vi "DTC_PERSISTANT.vi"(8 "errin":errorcluster, 11 "UNINIT?":bool) -> (0 "error out":errorcluster, 3 "Erased?":bool)   [LabVIEW 2020]
uses:
  <userlib>/PCAN Basic/Controls/BaudrateEenum.ctl
  <userlib>/PCAN Basic/Controls/Channel.ctl
  41182dc3-e488-4534-8057-e389c647f1e6.vi
  OP500/VG/VG_branche.vi
  <userlib>/Alex_Peak_lib/PEAK_lib_ALEX.lvlib
  <userlib>/PCAN Basic/PCANBasic.lvlib
panel:
  out "dataout":T1 {"ID" format="%.0x"}
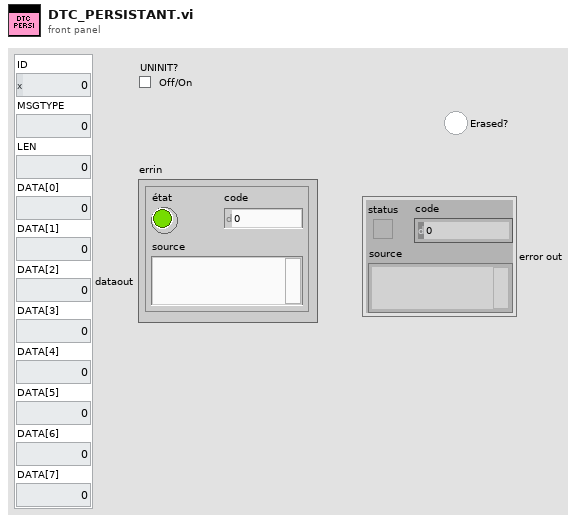
[diagram p1: front panel]
types:
  T1 = cluster{"ID":u32, "MSGTYPE":u8, "LEN":u8, "DATA[0]":u8, "DATA[1]":u8, "DATA[2]":u8, "DATA[3]":u8, "DATA[4]":u8, "DATA[5]":u8, "DATA[6]":u8, "DATA[7]":u8}
  T2 = typedef "PCANBasic.lvlib/Channel.ctl" = enum16{"PCAN_NONEBUS", "not used1", "not used2", "not used3", "not used4", "not used5", "not used6", "not used7", "not used8", "not used9", "not used10", "not used11", "not used12", "not used13", "not used14", "not used15", "not used16", "not used17", "not used18", "not used19", "not used20", "not used21", "not used22", "not used23", "not used24", "not used25", "not used26", "not used27", "not used28", "not used29", "not used30", "not used31", "not used32", "PCAN_ISABUS1", "PCAN_ISABUS2", "PCAN_ISABUS3", "PCAN_ISABUS4", "PCAN_ISABUS5", "PCAN_ISABUS6", "PCAN_ISABUS7", "PCAN_ISABUS8", "not used41", "not used42", "not used43", "not used44", "not used45", "not used46", "not used47", "not used48", "PCAN_DNGBUS1", "not used50", "not used51", "not used52", "not used53", "not used54", "not used55", "not used56", "not used57", "not used58", "not used59", "not used60", "not used61", "not used62", "not used63", "not used64", "PCAN_PCIBUS1", "PCAN_PCIBUS2", "PCAN_PCIBUS3", "PCAN_PCIBUS4", "PCAN_PCIBUS5", "PCAN_PCIBUS6", "PCAN_PCIBUS7", "PCAN_PCIBUS8", "not used73", "not used74", "not used75", "not used76", "not used77", "not used78", "not used79", "not used80", "PCAN_USBBUS1", "PCAN_USBBUS2", "PCAN_USBBUS3", "PCAN_USBBUS4", "PCAN_USBBUS5", "PCAN_USBBUS6", "PCAN_USBBUS7", "PCAN_USBBUS8", "Not used89", "Not used90", "Not used91", "Not used92", "Not used93", "Not used94", "Not used95", "Not used96", "PCAN_PCCBUS1", "PCAN_PCCBUS2"}
  T3 = typedef "PCANBasic.lvlib/BaudrateEenum.ctl" = enum16{"CAN_Baud_1M", "CAN_Baud_800K", "CAN_BAUD_500K", "CAN_BAUD_250K", "CAN_BAUD_125K", "CAN_BAUD_100K", "CAN_BAUD_95K", "CAN_BAUD_83K", "CAN_BAUD_50K", "CAN_BAUD_47K", "CAN_BAUD_33K", "CAN_BAUD_20K", "CAN_BAUD_10K", "CAN_BAUD_5K", "User Baudrate"}
  T4 = cluster{"ID":u32, "MSGTYPE":u8, "LEN":u8, "DATA[0]":ext, "DATA[1]":ext, "DATA[2]":ext, "DATA[3]":ext, "DATA[4]":ext, "DATA[5]":ext, "DATA[6]":ext, "DATA[7]":ext}
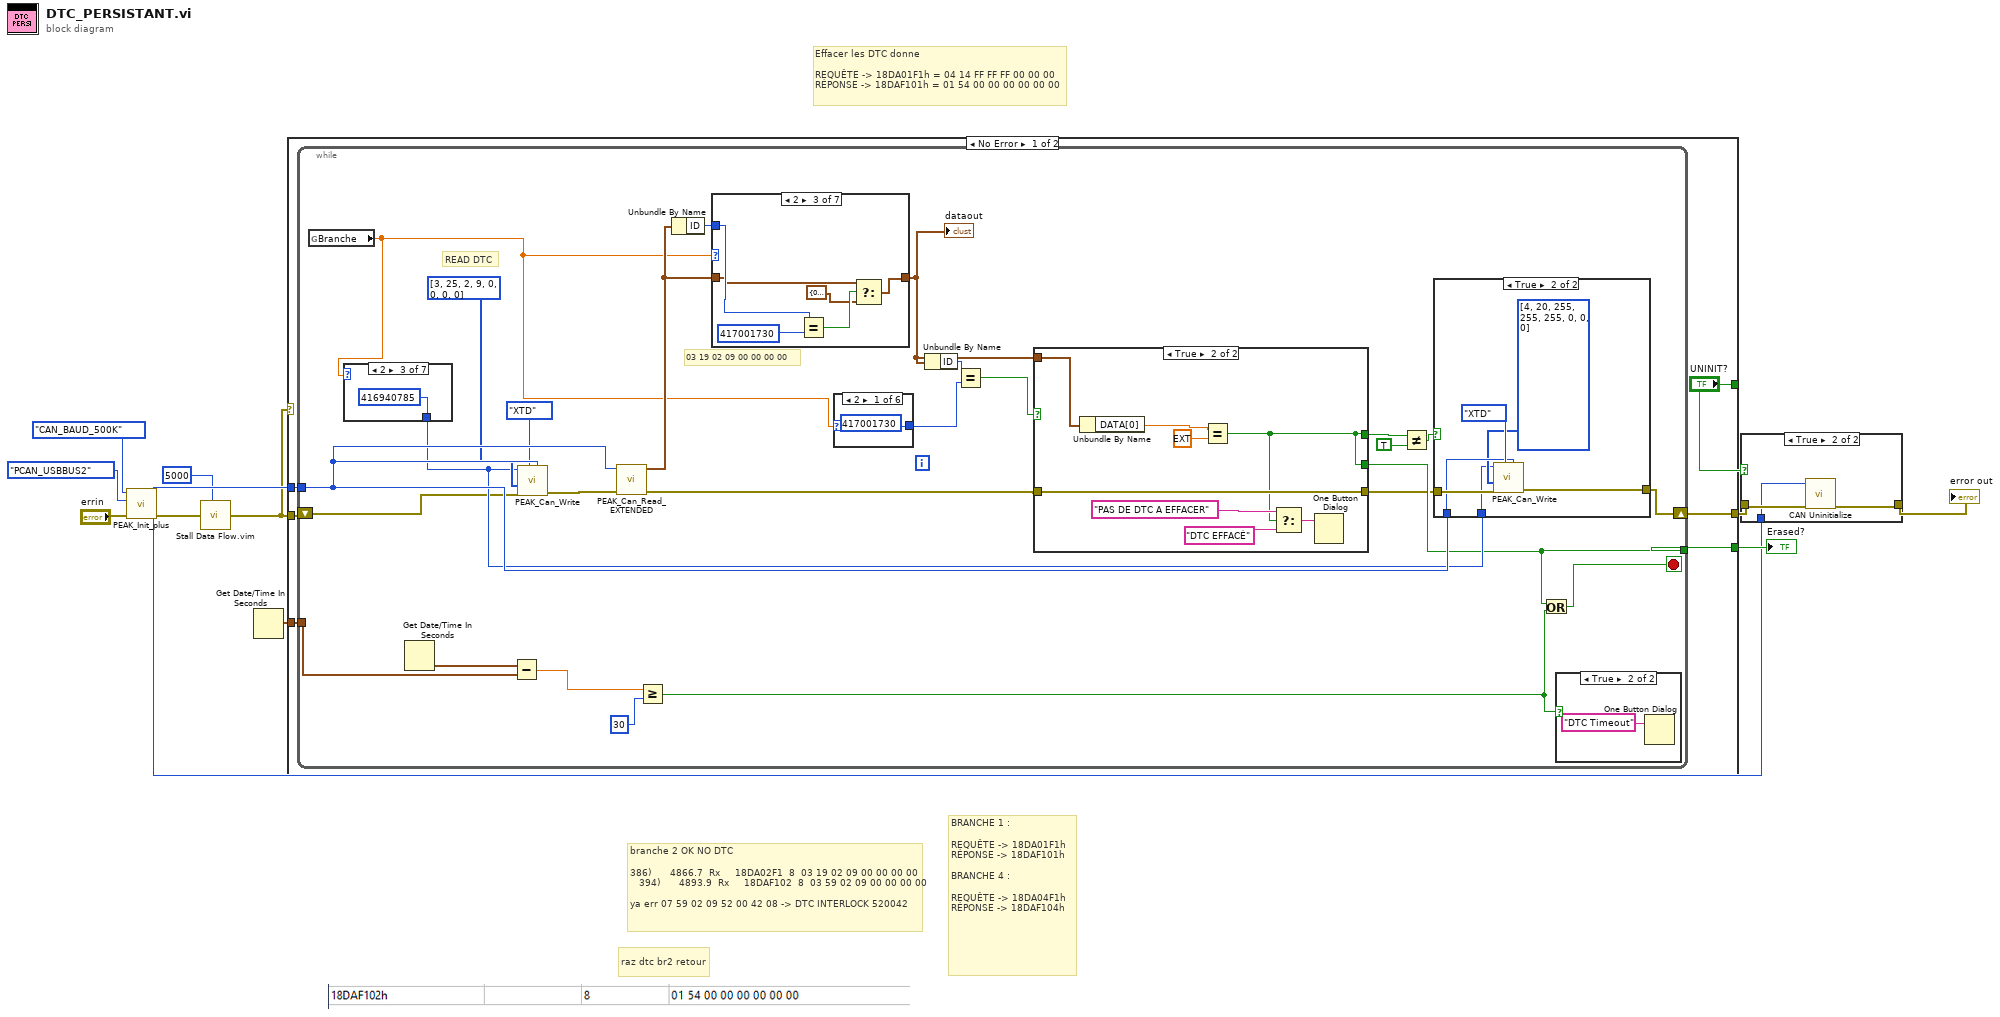
[diagram p0: block diagram]
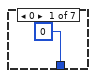
[diagram p2: hidden frame]
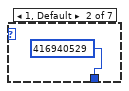
[diagram p3: hidden frame]
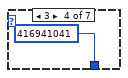
[diagram p4: hidden frame]
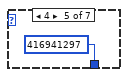
[diagram p5: hidden frame]
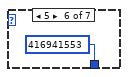
[diagram p6: hidden frame]
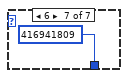
[diagram p7: hidden frame]
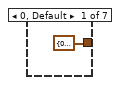
[diagram p8: hidden frame]
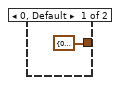
[diagram p10: hidden frame]
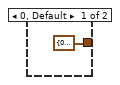
[diagram p12: hidden frame]
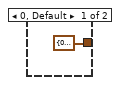
[diagram p14: hidden frame]
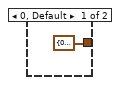
[diagram p16: hidden frame]
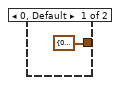
[diagram p18: hidden frame]
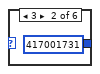
[diagram p19: hidden frame]
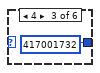
[diagram p20: hidden frame]
diagram:
  # "raz dtc br2 retour"
  # "branche 2 OK NO DTC\n\n386)      4866.7  Rx     18DA02F1  8  03 19 02 09 00 00 00 00 \n   394)      4893.9  Rx     18DAF102  8  03 59 02 09 00 00 00 00\n\nya err 07 59 02 09 52 00 42 08 -> DTC INTERLOCK 520042"
  # "BRANCHE 1 :\n\nREQUÊTE -> 18DA01F1h\nRÉPONSE -> 18DAF101h\n\nBRANCHE 4 :\n\nREQUÊTE -> 18DA04F1h\nRÉPONSE -> 18DAF104h"
  # "Effacer les DTC donne \n\nREQUÊTE -> 18DA01F1h = 04 14 FF FF FF 00 00 00\nRÉPONSE -> 18DAF101h = 01 54 00 00 00 00 00 00"
  n1 = call <userlib>:"PEAK_Init_plus.vi"("errin"="errin", "Channel"=Channel."PCAN_USBBUS2", "BTR0BTR1"=BaudrateEenum."CAN_BAUD_500K") -> ("errout"=w3:errorcluster, "Channel out"=w4:T2)  [unwired: 7 in]
  n2 = call "Stall Data Flow.vim"("value in"=w3, "milliseconds to wait"=u32 5000) -> ("value out"=w2:errorcluster)  [unwired: 1 out]
  n3 = Get Date/Time In Seconds() -> (seconds since 1Jan1904=w10:timestamp)
  n4 = case shown="No Error" w2 {
    tunnel: w2 -> [w18 w109]
    tunnel: [w17 _] -> w11
    tunnel: w10 -> [w16 _]
    tunnel: [w15 w109] -> w9
    tunnel: ["UNINIT?" FALSE ("UNINIT?")] -> w7
    tunnel: w4 -> [w13 _]
    frame No Error {
      n5 = while {
        tunnel: w13 -> [w41]
        shift-right: [w33] -> w15
        shift-left: w18 -> [w30]
        tunnel: [w28] -> w17
        tunnel: w16 -> [w27]
        stop <- w29 stop-if-true
        # "READ DTC"
        # "03 19 02 09 00 00 00 00"
        n6 = global read "VG_branche.vi" "Branche"() -> (w31:dbl)
        n7 = case shown="2" w31 {
          tunnel: [u32 0 ("Identifier") u32 416940529 ("Identifier") u32 416940785 ("Identifier") u32 416941041 ("Identifier") u32 416941297 ("Identifier") u32 416941553 ("Identifier") u32 416941809 ("Identifier")] -> w34
          frame 0 {
          }
          frame 1, Default {
          }
          frame 2 {
          }
          frame 3 {
          }
          frame 4 {
          }
          frame 5 {
          }
          frame 6 {
          }
        }
        n8 = Get Date/Time In Seconds() -> (seconds since 1Jan1904=w26:timestamp)
        n9 = Subtract(x=w26, y=w27) -> (x-y=w25:dbl)
        n10 = call <userlib>:"PEAK_Can_Write.vi"("CAN handle"=w41, "MSG type"=enum8{"STD", "RTR", "XTD", "XTD RTR", "STATUS"}."XTD", "errin"=w30, "CAN Data"=i32[] [3, 25, 2, 9, 0, 0, 0, 0], "Identifier"=w34) -> ("errout"=w19:errorcluster)  [unwired: 6 in]
        n11 = call <userlib>:"PEAK_Can_Read_EXTENDED.vi"("errin"=w19, "Channel out"=w41) -> ("errout"=w43:errorcluster, "MessageBuffer out"=w39:T4)  [unwired: 7 in, 1 out]
        n12 = Greater Or Equal?(x=w25, y=30) -> (x >= y?=w23:bool)
        n13 = Unbundle By Name(w39) -> ("ID"=w40:u32)
        n14 = case shown="2" w31 {
          tunnel: w40 -> [_ w55 w62 w66 w71 w76 w80]
          tunnel: w39 -> [_ w54 w59 w65 w70 w75 w81]
          tunnel: [T1 {"ID"=0, "MSGTYPE"=0, "LEN"=0, "DATA[0]"=0, "DATA[1]"=0, "DATA[2]"=0, "DATA[3]"=0, "DATA[4]"=0, "DATA[5]"=0, "DATA[6]"=0, "DATA[7]"=0} ("MessageBuffer out") w53 w58 w64 w69 w74 w79] -> w44
          frame 0, Default {
          }
          frame 1 {
            # "Fonction branche"
            n15 = case shown="18DAF101" w55 {
              tunnel: w54 -> [_ w57]
              tunnel: [T1 {"ID"=0, "MSGTYPE"=0, "LEN"=0, "DATA[0]"=0, "DATA[1]"=0, "DATA[2]"=0, "DATA[3]"=0, "DATA[4]"=0, "DATA[5]"=0, "DATA[6]"=0, "DATA[7]"=0} ("MessageBuffer out") w57] -> w53
              frame 0, Default {
              }
              frame 417001729 {
              }
            }
          }
          frame 2 {
            n16 = Equal?(x=w62, y=417001730) -> (x = y?=w61:bool)
            n17 = Select(t=w59, s=w61, f=T1 {"ID"=0, "MSGTYPE"=0, "LEN"=0, "DATA[0]"=0, "DATA[1]"=0, "DATA[2]"=0, "DATA[3]"=0, "DATA[4]"=0, "DATA[5]"=0, "DATA[6]"=0, "DATA[7]"=0} ("MessageBuffer out")) -> (s? t:f=w58:T4)
          }
          frame 3 {
            n18 = case shown="18DAF103" w66 {
              tunnel: w65 -> [_ w68]
              tunnel: [T1 {"ID"=0, "MSGTYPE"=0, "LEN"=0, "DATA[0]"=0, "DATA[1]"=0, "DATA[2]"=0, "DATA[3]"=0, "DATA[4]"=0, "DATA[5]"=0, "DATA[6]"=0, "DATA[7]"=0} ("MessageBuffer out") w68] -> w64
              frame 0, Default {
              }
              frame 417001731 {
              }
            }
          }
          frame 4 {
            n19 = case shown="18DAF104" w71 {
              tunnel: w70 -> [_ w73]
              tunnel: [T1 {"ID"=0, "MSGTYPE"=0, "LEN"=0, "DATA[0]"=0, "DATA[1]"=0, "DATA[2]"=0, "DATA[3]"=0, "DATA[4]"=0, "DATA[5]"=0, "DATA[6]"=0, "DATA[7]"=0} ("MessageBuffer out") w73] -> w69
              frame 0, Default {
              }
              frame 417001732 {
              }
            }
          }
          frame 5 {
            n20 = case shown="18DAF105" w76 {
              tunnel: w75 -> [_ w78]
              tunnel: [T1 {"ID"=0, "MSGTYPE"=0, "LEN"=0, "DATA[0]"=0, "DATA[1]"=0, "DATA[2]"=0, "DATA[3]"=0, "DATA[4]"=0, "DATA[5]"=0, "DATA[6]"=0, "DATA[7]"=0} ("MessageBuffer out") w78] -> w74
              frame 0, Default {
              }
              frame 417001733 {
              }
            }
          }
          frame 6 {
            n21 = case shown="18DAF106" w80 {
              tunnel: [T1 {"ID"=0, "MSGTYPE"=0, "LEN"=0, "DATA[0]"=0, "DATA[1]"=0, "DATA[2]"=0, "DATA[3]"=0, "DATA[4]"=0, "DATA[5]"=0, "DATA[6]"=0, "DATA[7]"=0} ("MessageBuffer out") w83] -> w79
              tunnel: w81 -> [_ w83]
              frame 0, Default {
              }
              frame 417001734 {
              }
            }
          }
        }
        "dataout" <- w44
        n22 = case shown="2" w31 {
          tunnel: [417001730 417001731 417001732 417001733 417001734 417001729] -> w35
          frame 2 {
          }
          frame 3 {
          }
          frame 4 {
          }
          frame 5 {
          }
          frame 6 {
          }
          frame 1, Default {
          }
        }
        n23 = Unbundle By Name(w44) -> ("ID"=w36:u32)
        n24 = Equal?(x=w36, y=w35) -> (x = y?=w20:bool)
        n25 = case shown="True" w20 {
          tunnel: w44 -> [_ w95]
          tunnel: [w90 w92] -> w42
          tunnel: [w91 w98] -> w22
          tunnel: w43 -> [w91 w98]
          tunnel: [w90 w92] -> w28
          frame False {
            w90 = FALSE
          }
          frame True {
            n26 = Unbundle By Name(w95) -> ("DATA[0]"=w94:ext)
            n27 = Equal?(x=w94, y=ext 3.0) -> (x = y?=w92:bool)
            n28 = Select(t="PAS DE DTC A EFFACER", s=w92, f="DTC EFFACÉ") -> (s? t:f=w96:string)
            n29 = One Button Dialog(message=w96) -> ()  [unwired: 1 in, 1 out]
          }
        }
        n30 = Not Equal?(x=w42, y=TRUE) -> (x != y?=w21:bool)
        n31 = case shown="True" w21 {
          tunnel: w22 -> [w100 w104]
          tunnel: w41 -> [_ w103]
          tunnel: w34 -> [_ w101]
          tunnel: [w100 w105] -> w33
          frame False {
          }
          frame True {
            n32 = call <userlib>:"PEAK_Can_Write.vi"("CAN handle"=w103, "MSG type"=enum8{"STD", "RTR", "XTD", "XTD RTR", "STATUS"}."XTD", "errin"=w104, "CAN Data"=i32[] [4, 20, 255, 255, 255, 0, 0, 0], "Identifier"=w101) -> ("errout"=w105:errorcluster)  [unwired: 6 in]
          }
        }
        n33 = Or(x=w28, y=w23) -> (x .or. y?=w29:bool)
        n34 = case shown="True" w23 {
          frame False {
          }
          frame True {
            n35 = One Button Dialog(message="DTC Timeout") -> ()  [unwired: 1 in, 1 out]
          }
        }
      }
    }
    frame Error {
    }
  }
  "Erased?" <- w11
  n36 = case shown="True" w7 {
    tunnel: w9 -> [w110 w113]
    tunnel: [w110 w112] -> w8
    tunnel: w4 -> [_ w111]
    frame False {
    }
    frame True {
      n37 = call <userlib>:"CAN Uninitialize.vi"("error in (no error)"=w113, "Channel"=w111) -> ("error out"=w112:errorcluster)  [unwired: 7 in, 2 out]
    }
  }
  "error out" <- w8
